vi "Create ToolstripLabel.vi"(7 "ImageIndex":i32, 8 "error in (no error)":errorcluster caption="错误输入（无错误）", 9 "Width":i32=100, 10 "text":string, 11 "StatusStripClass 输入":refnum<class "StatusStripClass.lvclass"> caption="DNL_LabVIEW Object in") -> (0 "error out":errorcluster caption="错误输出", 2 "ToolStripLabel 输出":refnum<class "ToolStripLabel.lvclass"> caption="DNL_LabVIEW Object out", 3 "StatusStripClass 输出":refnum<class "StatusStripClass.lvclass"> caption="DNL_LabVIEW Object out")   [LabVIEW 2013, in "StatusStripClass.lvclass"]
uses:
  StatusStripClass.lvclass
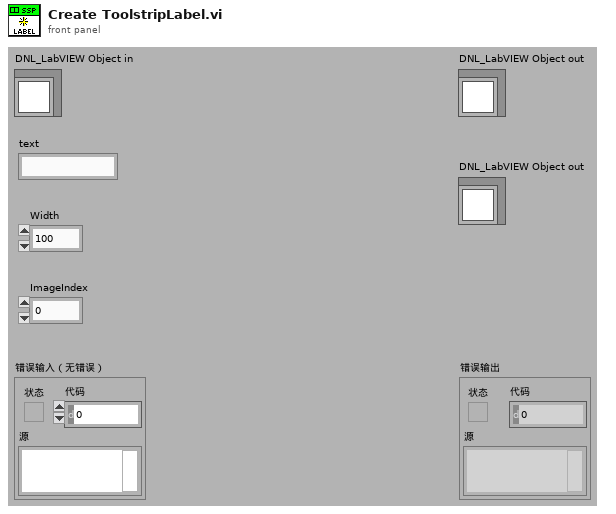
[diagram p1: front panel]
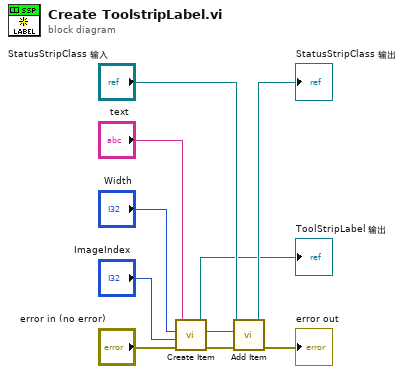
[diagram p0: block diagram]
diagram:
  n1 = call "Create Item.vi"("error in (no error)"="error in (no error)", "ImageIndex"="ImageIndex", "Width"="Width", "text"="text") -> ("error out"=w1:errorcluster, "ItemRef"=w10:refnum<k24>, "ToolStripLabel 输出"=→"ToolStripLabel 输出":refnum<class "ToolStripLabel.lvclass">)  [unwired: 5 in]
  n2 = call "Add Item.vi"("error in (no error)"=w1, "ItemRef"=w10, "StatusStripClass 输入"="StatusStripClass 输入") -> ("error out"=→"error out":errorcluster, "StatusStripClass 输出"=→"StatusStripClass 输出":refnum<class "StatusStripClass.lvclass">)  [unwired: 7 in]
